vi "get Area.vi"(10 "Laser":dbl, 11 "Cell Data Cluster":T1) -> (3 "Area":dbl)   [LabVIEW 2012]
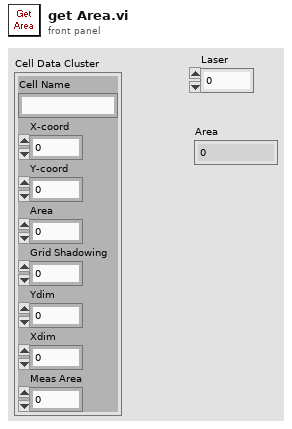
[diagram p1: front panel]
types:
  T1 = cluster{"Cell Name":string, "X-coord":dbl, "Y-coord":dbl, "Area":dbl, "Grid Shadowing":dbl, "Ydim":dbl, "Xdim":dbl, "Meas Area":dbl}
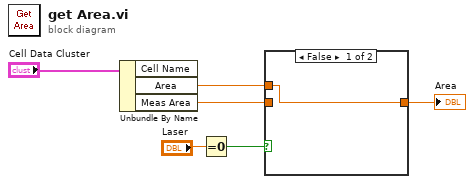
[diagram p0: block diagram]
diagram:
  n1 = Unbundle By Name("Cell Data Cluster") -> ("Area"=w1:dbl, "Meas Area"=w3:dbl)  [unwired: 1 out]
  n2 = Equal To 0?(x="Laser") -> (x = 0?=w4:bool)
  n3 = case shown="False" w4 {
    tunnel: w3 -> [_ w8]
    tunnel: [w7 w8] -> w2
    tunnel: w1 -> [w7 _]
    frame False {
    }
    frame True {
    }
  }
  "Area" <- w2
